vi "Save_data_txt.vi"(8 "error in (no error)":errorcluster, 10 "Grafica":waveform(dbl)(graph), 11 "Logging_tdms in":refnum<class "Logging_tdms.lvclass">) -> (0 "error out":errorcluster, 3 "Logging_txt out":refnum<class "Logging_txt.lvclass">)   [LabVIEW 2019, in "Logging_tdms.lvlib" / "Logging_tdms.lvclass"]
uses:
  Logging_tdms.lvclass
  C:/Users/Luis/Documents/Ingenieria/Git_versiones/Actor-framework-CML-con-opciones-de-adquisici-n-main/Logging_txt/Logging_txt/Logging_txt.lvclass
  Logging_txt/Logging_txt/Logging_txt.lvclass
  Logging_txt/Logging_txt/Logging_txt.lvclass/Logging_txt.ctl
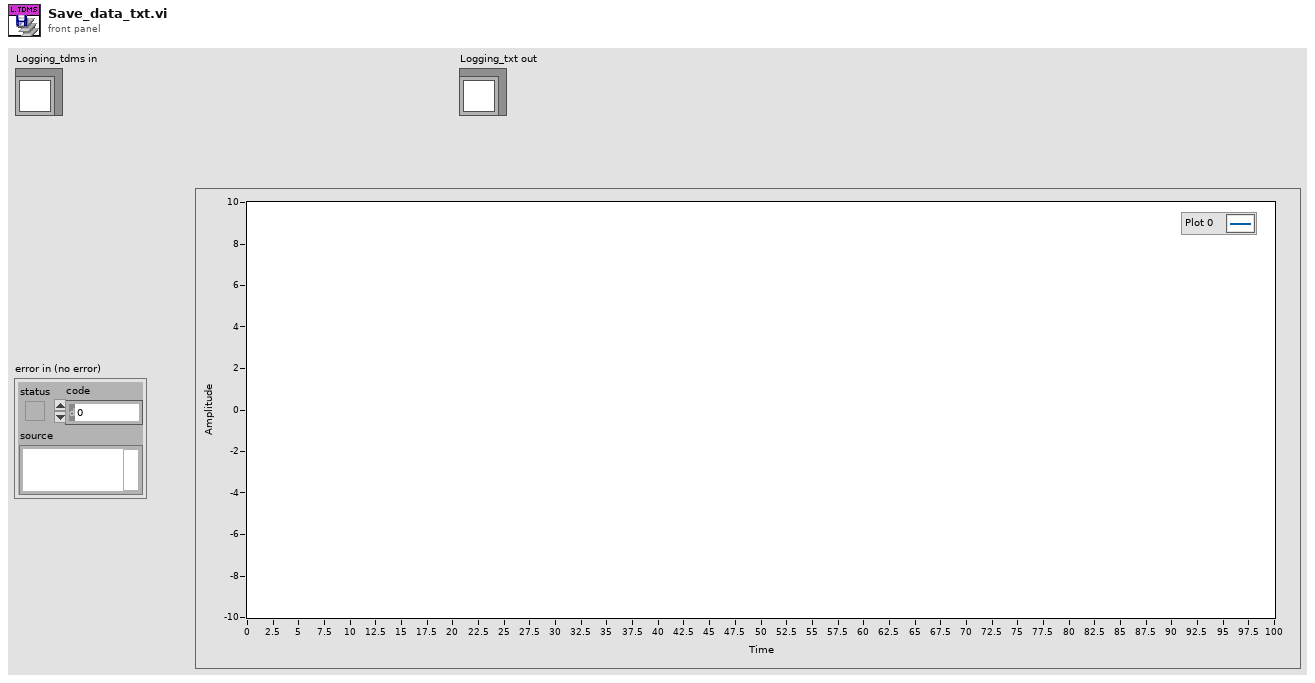
[diagram p1: front panel]
types:
  T1 = enum16{"open", "open or create", "create or replace", "create", "open (read-only)"}
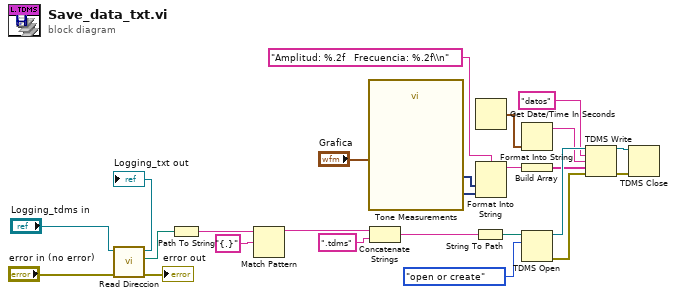
[diagram p0: block diagram]
diagram:
  n1 = call "Read Direccion.vi"("error in (no error)"="error in (no error)", "Logging_txt in"="Logging_tdms in") -> ("error out"=→"error out":errorcluster, "Direccion"=w17:path, "Logging_txt out"=→"Logging_txt out":refnum<class "Logging_tdms.lvclass">)  [unwired: 7 in]
  n2 = Path To String(path=w17) -> (string=w22:string)
  n3 = Match Pattern(string=w22, regular expression="{.}") -> (before substring=w20:string)  [unwired: 1 in, 3 out]
  n4 = call "Tone Measurements"("Signals"="Grafica") -> ("Frequency"=w8:dynamicdata, "Amplitude"=w7:dynamicdata)  [unwired: 8 in, 1 out]
  n5 = Concatenate Strings(w20, ".tdms" ("string")) -> (w18:string)
  n6 = String To Path(string=w18) -> (path=w6:path)
  n7 = Get Date/Time In Seconds() -> (seconds since 1Jan1904=w10:timestamp)
  n8 = Format Into String(format string="Amplitud: %.2f   Frecuencia: %.2f\\n", w7, w8) -> (resulting string=w3:string)  [unwired: 2 in, 1 out]
  n9 = Format Into String(w10) -> (resulting string=w1:string)  [unwired: 3 in, 1 out]
  n10 = Build Array(w3) -> (w2:string[])
  n11 = TDMS Open(10:T1."open or create" ("operation (0:open)"), 11:w6) -> (0:w12:errorcluster, 3:w13:refnum<k34>)  [unwired: 5 in]
  n12 = TDMS Write(0:w13, 5:"datos" ("group name in (Untitled)"), 7:w1, 9:w2, 11:w12) -> (4:w14:refnum<k34>, 15:w15:errorcluster)  [unwired: 1 in, 2 out]
  n13 = TDMS Close(8:w15, 11:w14) -> ()  [unwired: 2 out]
